vi "线下管理程序.vi"() -> ()   [LabVIEW 2013]
uses:
  <vilib>/Utility/error.llb/whitespace.ctl
panel:
  in  "生产":bool
  out "阻挡":bool
  in  "换工装":bool
  out "放行":bool
  in  "随形板ID":string
  in  "条码查询":bool
  in  "条码查询1":string
  in  "写入条码":bool
  in  "删除按钮":bool
  in  "删除条码":string
  in  "写入条码1":string
  out "Table 2":string[][](table) caption="RFID管理"
  in  "B020锁定":bool
  in  "B010锁定":bool
  in  "合格":bool
  in  "要写入的壳体条码":string
  out "error out":errorcluster
  out "Table":string[][](table) caption="B030数据库"
  in  "B020解除不合格":bool
  in  "B010解除不合格":bool
  in  "写入合格":bool
  in  "查询壳体条码":bool
  in  "壳体条码":string
  out "B020有不合格项":bool
  out "B020有不合格项":bool
  out "B020状态正常":bool
  out "B010状态正常":bool
  # "B030管理程序"
  # "B020状态"
  # "B010状态"
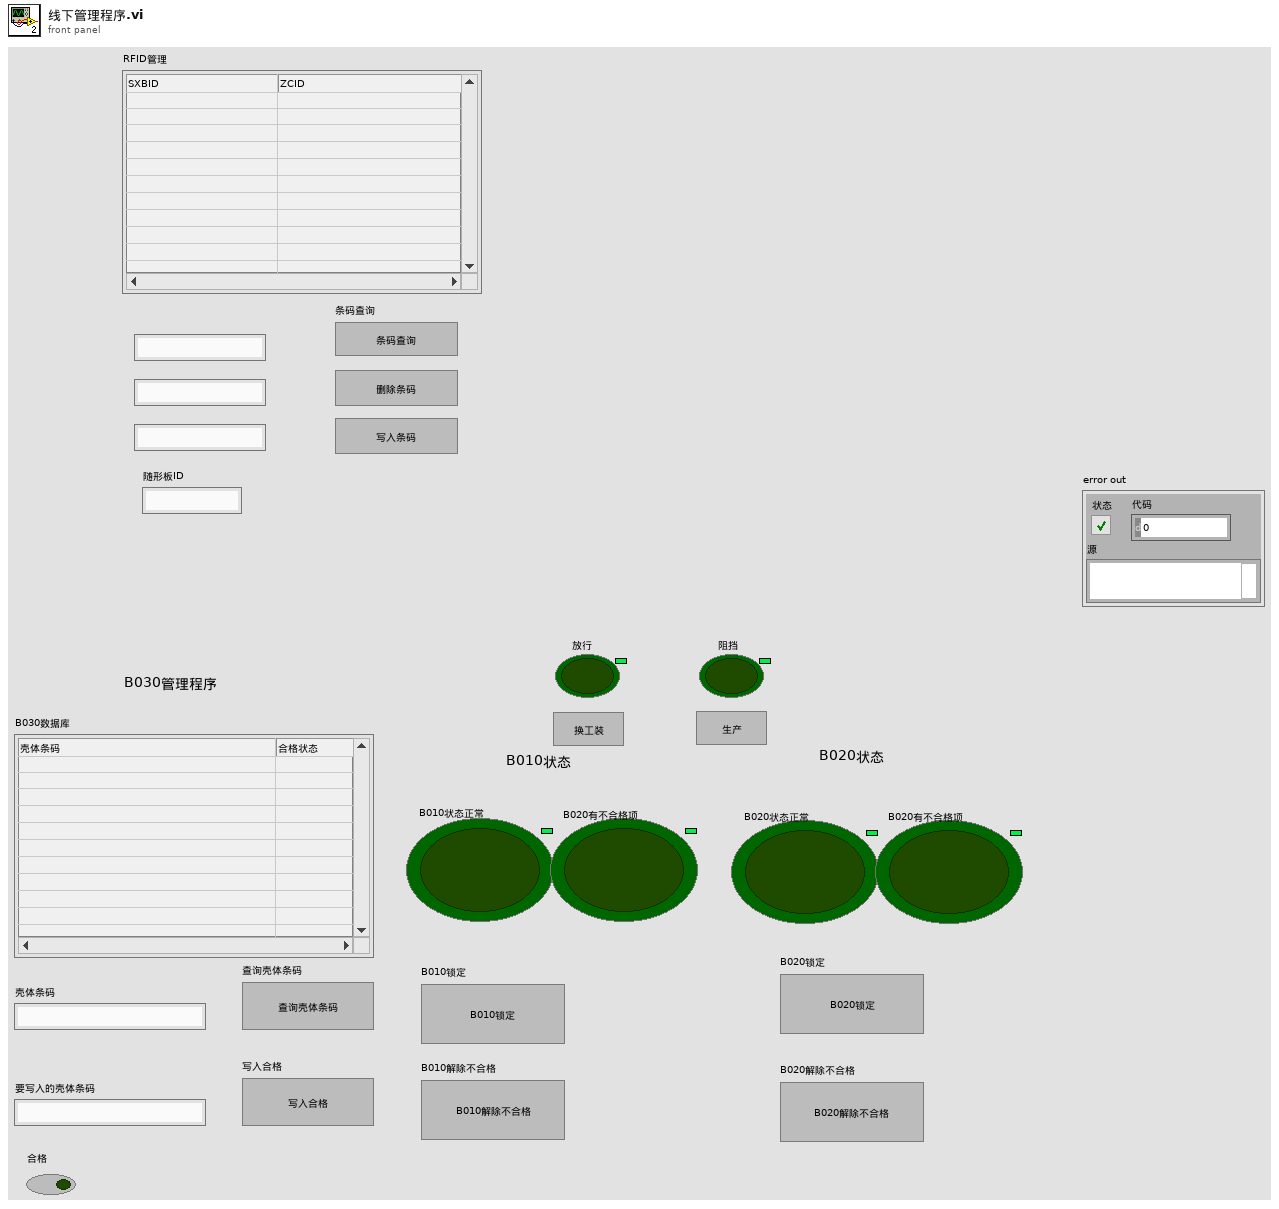
[diagram p1: front panel]
types:
  T1 = typedef "LVRowAndColumnTypeDef.ctl" = cluster{"Row":i32, "Column":i32}
  T2 = typedef "whitespace.ctl" = u16
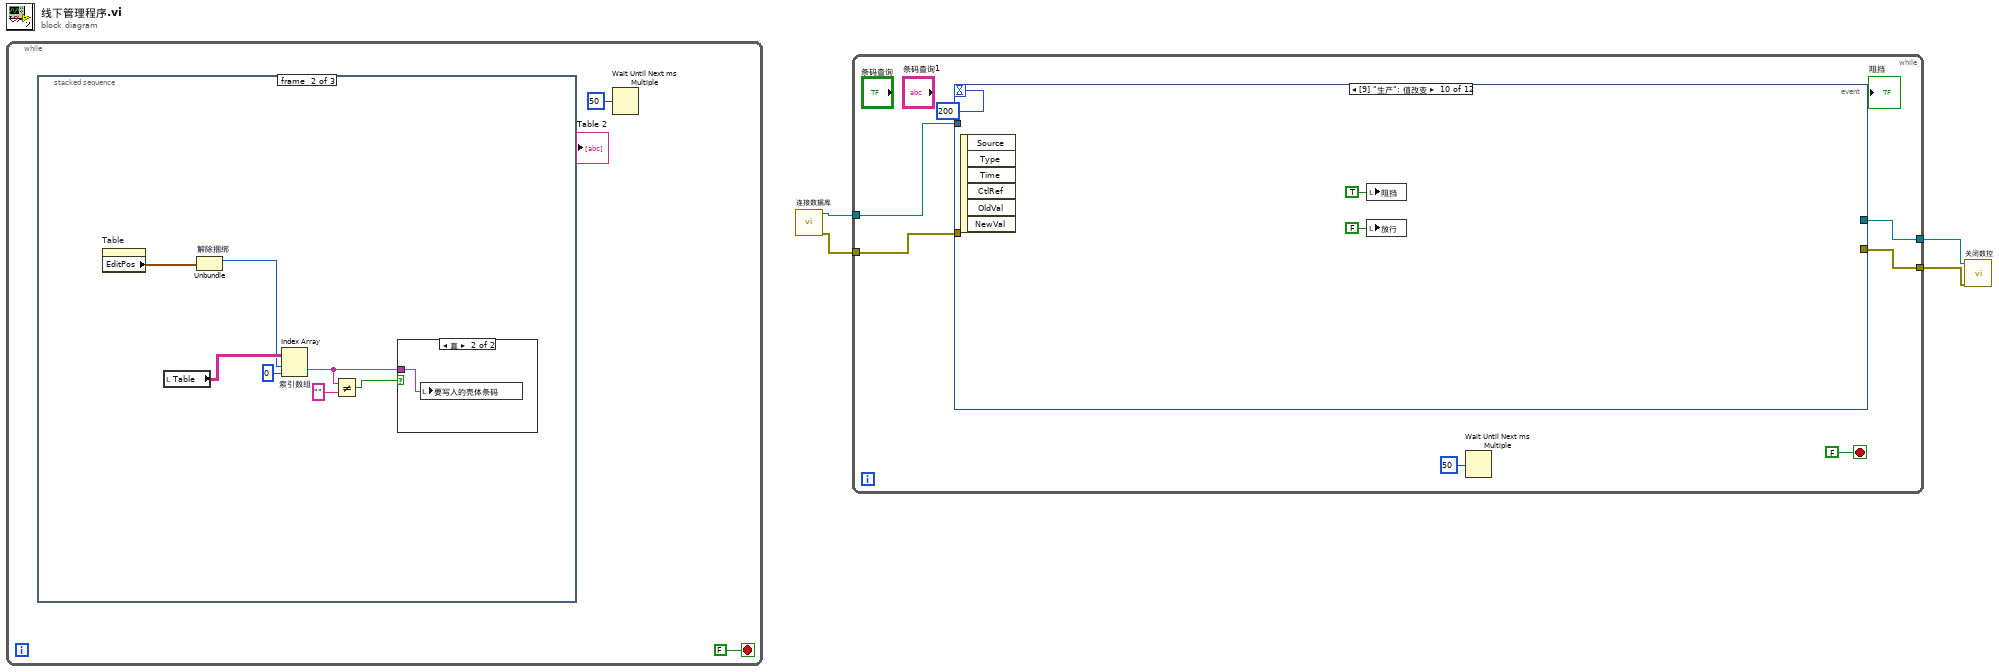
[diagram p0: block diagram]
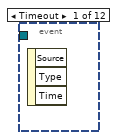
[diagram p2: hidden frame]
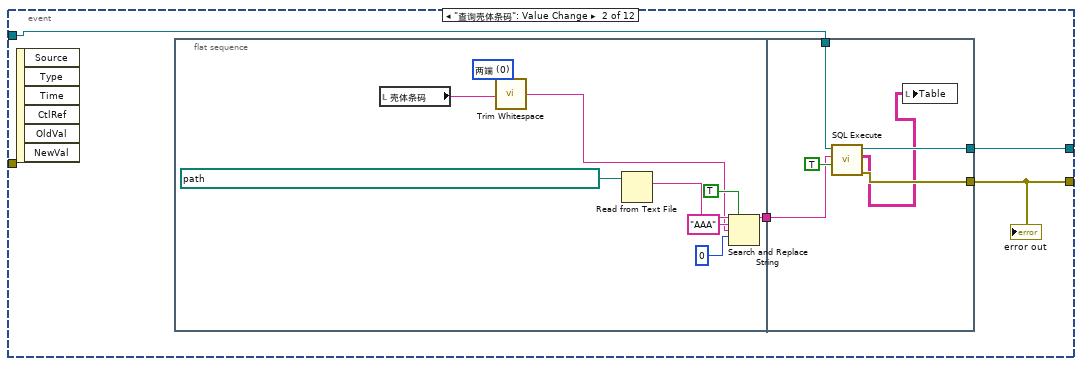
[diagram p3: hidden frame]
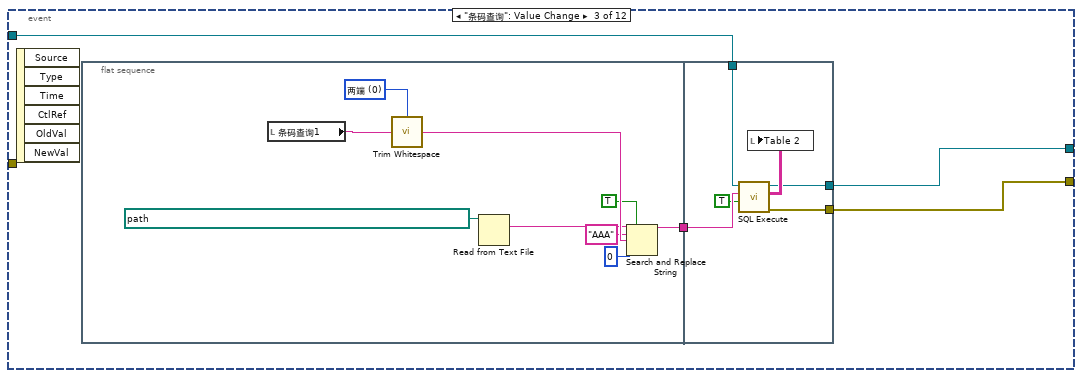
[diagram p4: hidden frame]
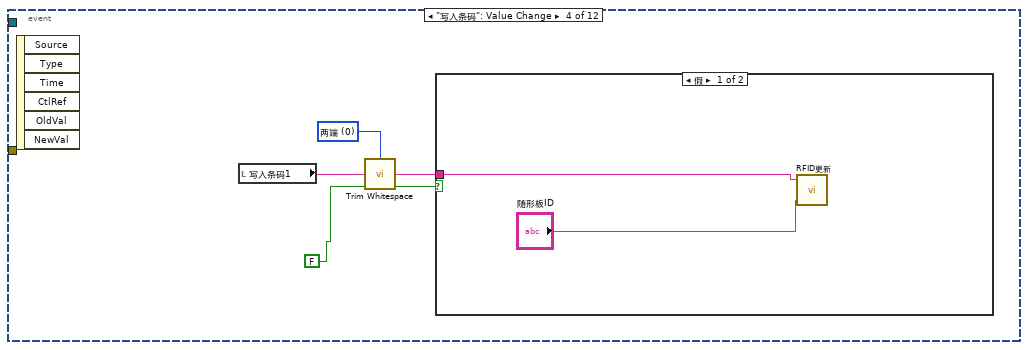
[diagram p5: hidden frame]
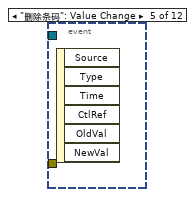
[diagram p7: hidden frame]
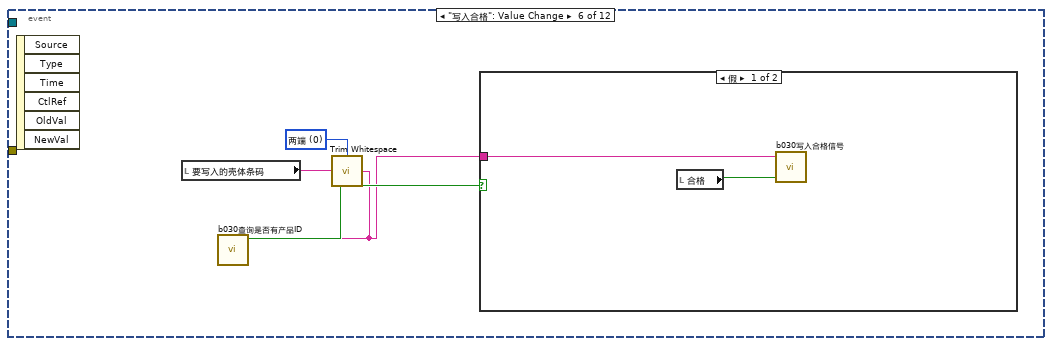
[diagram p8: hidden frame]
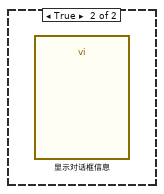
[diagram p9: hidden frame]
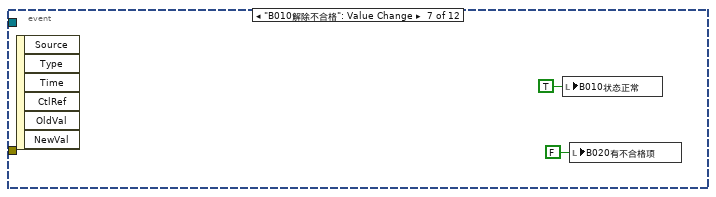
[diagram p10: hidden frame]
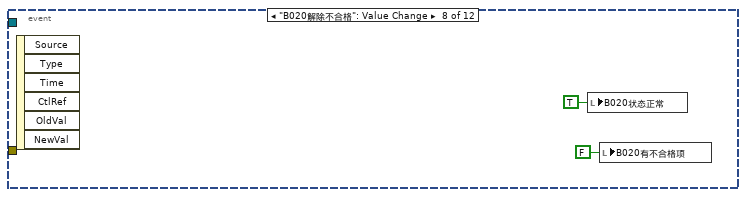
[diagram p11: hidden frame]
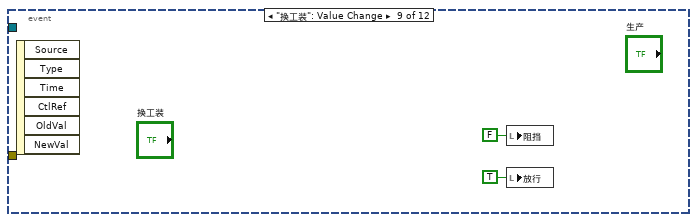
[diagram p12: hidden frame]
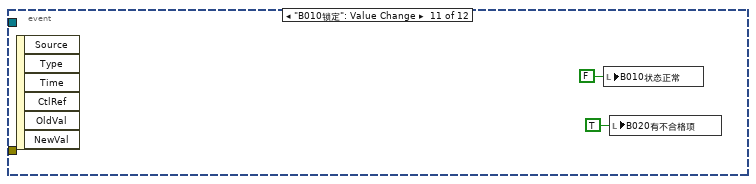
[diagram p13: hidden frame]
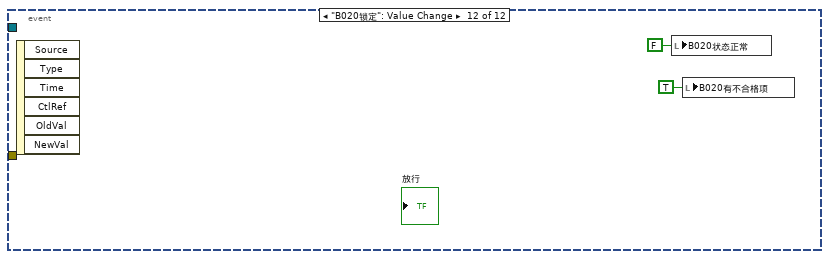
[diagram p14: hidden frame]
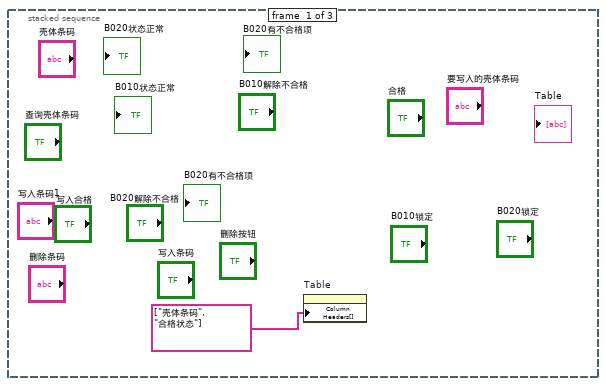
[diagram p15: hidden frame]
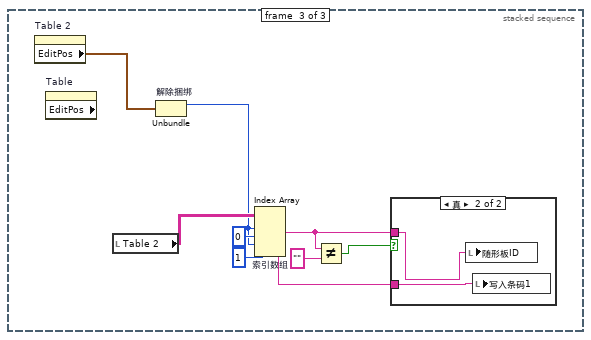
[diagram p17: hidden frame]
diagram:
  n1 = while {
    stop <- FALSE stop-if-true
    n2 = stacked-sequence {
      frame #0 {
        n3 = property on="Table" class="Tbl (严格)"("Column Headers[]"=string[] ["壳体条码", "合格状态"] ("行首字符串[]")) -> ()  [unwired: 2 in, 2 out]
      }
      frame #1 {
        n4 = property on="Table" class="Tbl (严格)"() -> ("EditPos"=w14:T1)  [unwired: 2 in, 2 out]
        n5 = local read "Table"() -> (w13:string[][])
        n6 = Unbundle "解除捆绑"(w14) -> ("Row"=w11:i32)  [unwired: 1 out]
        n7 = Index Array "索引数组"(array=w13, index (row)=w11, index (col)=0 ("禁用的索引 (列)")) -> (element=w8:string)
        n8 = Not Equal?(x=w8, y="") -> (x != y?=w9:bool)
        n9 = case shown="真" w9 {
          tunnel: w8 -> [_ w15]
          frame False {
          }
          frame True {
            n10 = local write "要写入的壳体条码"(w15) -> ()
          }
        }
      }
      frame #2 {
        n11 = property on="Table 2" class="Tbl (严格)"() -> ("EditPos"=w19:T1)  [unwired: 2 in, 2 out]
        n12 = property on="Table" class="Tbl (严格)" props=["EditPos"]() -> ()  [unwired: 2 in, 3 out]
        n13 = local read "Table 2"() -> (w24:string[][])
        n14 = Unbundle "解除捆绑"(w19) -> ("Row"=w18:i32)  [unwired: 1 out]
        n15 = Index Array "索引数组"(array=w24, index (row) #1=w18, index (col) #1=0 ("禁用的索引 (列)"), index (row) #2=w18, index (col) #2=1 ("禁用的索引 (列)")) -> (element #1=w20:string, element #2=w16:string)
        n16 = Not Equal?(x=w20, y="") -> (x != y?=w21:bool)
        n17 = case shown="真" w21 {
          tunnel: w20 -> [_ w26]
          tunnel: w16 -> [_ w25]
          frame False {
          }
          frame True {
            n18 = local write "随形板ID"(w26) -> ()
            n19 = local write "写入条码1"(w25) -> ()
          }
        }
      }
    }
    n20 = Wait Until Next ms Multiple(millisecond multiple=u32 50 ("毫秒倍数")) -> ()  [unwired: 1 out]
  }
  n21 = call "连接数据库.vi"() -> ("error out"=w3:errorcluster, "ADODB._Connection Out"=w4:refnum<k7>)  [unwired: 10 in]
  n22 = while {
    tunnel: w4 -> [w30]
    tunnel: w3 -> [w29]
    tunnel: [w28] -> w2
    tunnel: [w27] -> w1
    stop <- FALSE stop-if-true
    n23 = event shown="[9] \"生产\": 值改变" {
      selector: _ -> [_ _ _ _ _ _ _ _ _ _ _ _]
      dyn-events: _ -> [_ _ _ _ _ _ _ _ _ _ _ _]
      timeout: 200 -> [_ _ _ _ _ _ _ _ _ _ _ _]
      tunnel: w30 -> [_ w37 w56 _ _ _ _ _ _ _ _ _]
      tunnel: w29 -> [_ _ _ _ _ _ _ _ _ _ _ _]
      tunnel: [_ w35 w54 _ _ _ _ _ _ _ _ _] -> w28
      tunnel: [_ w34 w53 _ _ _ _ _ _ _ _ _] -> w27
      event Timeout {
        n24 = event-data() -> ()  [unwired: 1 in, 3 out]
      }
      event "查询壳体条码": Value Change {
        n25 = event-data() -> ()  [unwired: 1 in, 6 out]
        n26 = flat-sequence {
          tunnel: [w38] -> w36
          tunnel: w37 -> [w51]
          tunnel: w36 -> [w50]
          tunnel: [w49] -> w35
          tunnel: [w48] -> w34
          frame #0 {
            w46 = T2 0 items=["两端", "字符串首端", "字符串末端"] ("location (both)")
            n27 = local read "壳体条码"() -> (w45:string)
            n28 = call <vilib>:"Trim Whitespace.vi"("string"=w45, "location (both)"=w46) -> ("trimmed string"=w39:string)
            n29 = Read from Text File(file (use dialog)=path "F:/Q14070/Q14070生产管理系统/线下管理子VI/b030壳体质量数据查询.txt" ("文件（使用对话框）")) -> (text=w42:string)  [unwired: 3 in, 3 out]
            n30 = Search and Replace String(replace all?=TRUE ("替换全部？(F)"), input string=w42, search string="AAA" ("搜索字符串"), replace string=w39, offset=0 ("偏移量(0)")) -> (result string=w38:string)  [unwired: 3 in, 3 out]
          }
          frame #1 {
            n31 = call "SQL Execute.vi"("Return Data (T)"=TRUE, "Command Text"=w50, "ADODB._Connection In"=w51) -> ("error out"=w48:errorcluster, "Data"=w47:string[][], "ADODB._Connection Out"=w49:refnum<k7>)  [unwired: 5 in, 1 out]
            n32 = local write "Table"(w47) -> ()
          }
        }
        "error out" <- w34
      }
      event "条码查询": Value Change {
        n33 = event-data() -> ()  [unwired: 1 in, 6 out]
        n34 = flat-sequence {
          tunnel: [w57] -> w55
          tunnel: w56 -> [w71]
          tunnel: w55 -> [w70]
          tunnel: [w67] -> w54
          tunnel: [w66] -> w53
          frame #0 {
            w63 = T2 0 items=["两端", "字符串首端", "字符串末端"] ("location (both)")
            n35 = local read "条码查询1"() -> (w64:string)
            n36 = call <vilib>:"Trim Whitespace.vi"("string"=w64, "location (both)"=w63) -> ("trimmed string"=w65:string)
            n37 = Read from Text File(file (use dialog)=path "F:/Q14070/Q14070生产管理系统/线下管理子VI/RFID操作.txt" ("文件（使用对话框）")) -> (text=w61:string)  [unwired: 3 in, 3 out]
            n38 = Search and Replace String(replace all?=TRUE ("替换全部？(F)"), input string=w61, search string="AAA" ("搜索字符串"), replace string=w65, offset=0 ("偏移量(0)")) -> (result string=w57:string)  [unwired: 3 in, 3 out]
          }
          frame #1 {
            n39 = call "SQL Execute.vi"("Return Data (T)"=TRUE, "Command Text"=w70, "ADODB._Connection In"=w71) -> ("error out"=w66:errorcluster, "Data"=w68:string[][], "ADODB._Connection Out"=w67:refnum<k7>)  [unwired: 5 in, 1 out]
            n40 = local write "Table 2"(w68) -> ()
          }
        }
      }
      event "写入条码": Value Change {
        w74 = T2 0 items=["两端", "字符串首端", "字符串末端"] ("location (both)")
        n41 = event-data() -> ()  [unwired: 1 in, 6 out]
        n42 = local read "写入条码1"() -> (w75:string)
        n43 = call <vilib>:"Trim Whitespace.vi"("string"=w75, "location (both)"=w74) -> ("trimmed string"=w73:string)
        n44 = case shown="假" FALSE {
          tunnel: w73 -> [w77 _]
          frame False {
            n45 = call "RFID更新.vi"("随形板ID"="随形板ID", "壳体码"=w77) -> ()  [unwired: 3 in]
          }
          frame True {
          }
        }
      }
      event "删除条码": Value Change {
        n46 = event-data() -> ()  [unwired: 1 in, 6 out]
      }
      event "写入合格": Value Change {
        w81 = T2 0 items=["两端", "字符串首端", "字符串末端"] ("location (both)")
        n47 = event-data() -> ()  [unwired: 1 in, 6 out]
        n48 = local read "要写入的壳体条码"() -> (w80:string)
        n49 = call <vilib>:"Trim Whitespace.vi"("string"=w80, "location (both)"=w81) -> ("trimmed string"=w78:string)
        n50 = call "b030查询是否有产品ID.vi"("转向器总成ID"=w78) -> ("无重号"=w79:bool)  [unwired: 9 in, 1 out]
        n51 = case shown="假" w79 {
          tunnel: w78 -> [w83 _]
          frame False {
            n52 = local read "合格"() -> (w82:bool)
            n53 = call "b030写入合格信号.vi"("信号"=w82, "产品ID"=w83) -> ()  [unwired: 3 in]
          }
          frame True {
            n54 = call "显示对话框信息"() -> ()  [unwired: 10 in, 2 out]
          }
        }
      }
      event "B010解除不合格": Value Change {
        n55 = event-data() -> ()  [unwired: 1 in, 6 out]
        n56 = local write "B010状态正常"(TRUE ("B010状态正常")) -> ()
        n57 = local write "B020有不合格项"(FALSE ("B020有不合格项")) -> ()
      }
      event "B020解除不合格": Value Change {
        n58 = event-data() -> ()  [unwired: 1 in, 6 out]
        n59 = local write "B020状态正常"(TRUE ("B020状态正常")) -> ()
        n60 = local write "B020有不合格项"(FALSE ("B020有不合格项")) -> ()
      }
      event "换工装": Value Change {
        n61 = event-data() -> ()  [unwired: 1 in, 6 out]
        n62 = local write "阻挡"(FALSE ("阻挡")) -> ()
        n63 = local write "放行"(TRUE ("放行")) -> ()
      }
      event "生产": Value Change {
        n64 = event-data() -> ()  [unwired: 1 in, 6 out]
        n65 = local write "阻挡"(TRUE ("阻挡")) -> ()
        n66 = local write "放行"(FALSE ("放行")) -> ()
      }
      event "B010锁定": Value Change {
        n67 = event-data() -> ()  [unwired: 1 in, 6 out]
        n68 = local write "B010状态正常"(FALSE ("B010状态正常")) -> ()
        n69 = local write "B020有不合格项"(TRUE ("B020有不合格项")) -> ()
      }
      event "B020锁定": Value Change {
        n70 = event-data() -> ()  [unwired: 1 in, 6 out]
        n71 = local write "B020状态正常"(FALSE ("B020状态正常")) -> ()
        n72 = local write "B020有不合格项"(TRUE ("B020有不合格项")) -> ()
      }
    }
    n73 = Wait Until Next ms Multiple(millisecond multiple=u32 50 ("毫秒倍数")) -> ()  [unwired: 1 out]
  }
  n74 = call "关闭数控.vi"("error in (no error)"=w1, "ADODB._Connection In"=w2) -> ()  [unwired: 9 in, 1 out]
